vi "GetLoopCounter.vi"(6 "error in":errorcluster, 9 "Loop in":refnum<class "Loop.lvclass">) -> (0 "error out":errorcluster, 3 "Loop out":refnum<class "Loop.lvclass">, 4 "counter UID":i32)   [LabVIEW 2014, in "Loop.lvclass"]
uses:
  Loop.lvclass
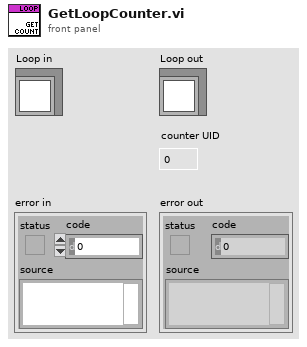
[diagram p1: front panel]
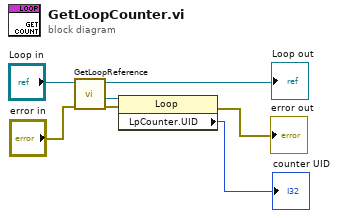
[diagram p0: block diagram]
diagram:
  n1 = call "GetLoopReference.vi"("error in"="error in", "Loop in"="Loop in") -> ("error out"=w4:errorcluster, "reference out"=w5:refnum<vi>, "Loop out"=→"Loop out":refnum<class "Loop.lvclass">)  [unwired: 7 in]
  n2 = property class="Loop"(reference=w5, error in=w4) -> (error out=→"error out":errorcluster, "LpCounter.UID"=→"counter UID":i32)  [unwired: 1 out]
